vi "print_to_console.vi"(8 "error in (no error)":errorcluster, 10 "log":T1 {"datetime" format="%<%x %.3X>T"}, 11 "console.provider in":refnum<class "console.provider.lvclass">) -> (0 "error out":errorcluster, 3 "console.provider out":refnum<class "console.provider.lvclass">)   [LabVIEW 2021, in "console.provider.lvclass"]
uses:
  console.provider.lvclass
  system.logging/log_entry.ctl
  system.logging/severity.ctl
  console_commands.ctl
  console_payload.ctl
  console.provider.lvclass/console.provider.ctl
  system.logging/system.logging.lvclass
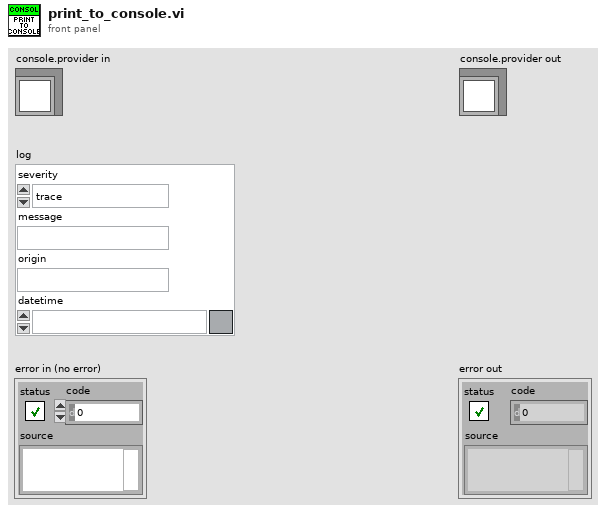
[diagram p1: front panel]
types:
  T1 = typedef "system.logging.lvclass/log_entry.ctl" = cluster{"severity":T2, "message":string, "origin":string, "datetime":timestamp}
  T2 = typedef "system.logging.lvclass/severity.ctl" = enum8{"trace", "debug", "info", "warning", "error"}
  T3 = typedef "console.provider.lvclass/console_commands.ctl" = enum16{"close", "print"}
  T4 = typedef "console.provider.lvclass/console_payload.ctl" = cluster{"console_cmd":T3, "log":T1}
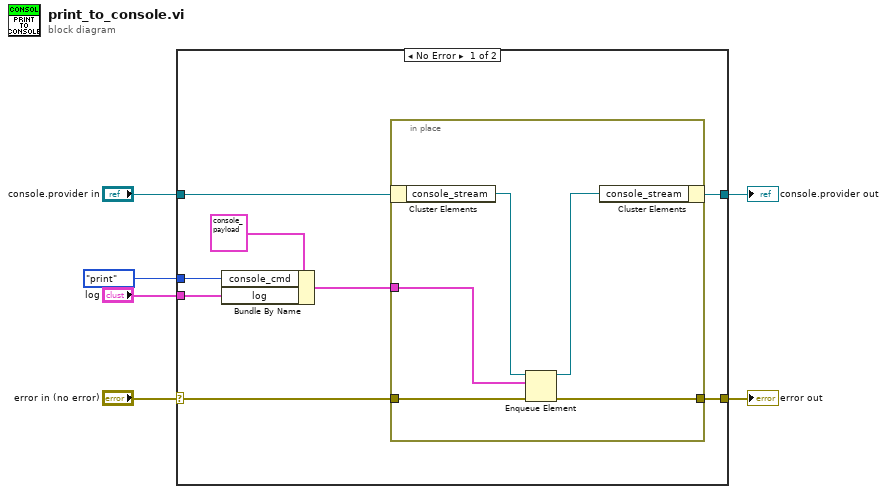
[diagram p0: block diagram]
diagram:
  n1 = case shown="No Error" "error in (no error)" {
    selector: "error in (no error)" -> [w13 w21]
    tunnel: [w11 w21] -> w5
    tunnel: [w12 w20] -> w3
    tunnel: "console.provider in" -> [w14 w20]
    tunnel: console_commands."print" ("console_cmd") -> [w9 _]
    tunnel: "log" -> [w8 _]
    frame No Error {
      n2 = Bundle By Name(cluster=T4 {"console_cmd"=enum."close", "log"={"severity"=enum."trace", "message"="", "origin"="", "datetime"=timestamp(0 s since 1904-01-01)}} ("console_payload"), "console_cmd"=w9, "log"=w8) -> (w7:T4)
      n3 = in-place {
        in-place-border: w13 -> [w19]
        in-place-border: [w16] -> w11
        in-place-border: w7 -> [w15]
        n4 = in-place-cluster #1(w14) -> ("console_stream"=w18:refnum<queue>)
        n5 = Enqueue Element(queue=w18, element=w15, error in (no error)=w19) -> (queue out=w17:refnum<queue>, error out=w16:errorcluster)  [unwired: 1 in, 1 out]
        n6 = in-place-cluster #1("console_stream"=w17) -> (w12:refnum<class "console.provider.lvclass">)
      }
    }
    frame Error {
    }
  }
  "error out" <- w5
  "console.provider out" <- w3
